vi "readPress02.vi"() -> ()   [LabVIEW 2011]
uses:
  Growth Sequences/Control 1.ctl
  <vilib>/Instr/_visa.llb/VISA Configure Serial Port (Instr).vi
panel:
  out "return count":u32
  in  "delay before read (ms)":u32=500
  in  "y":i32=1000
  in  "VISA resource name":T1="COM1"
  out "read buffer":string
  out "P (Torr)":dbl
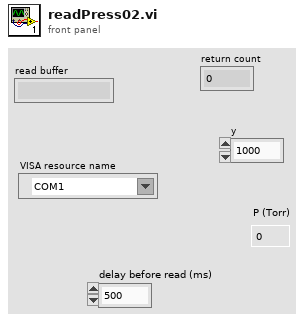
[diagram p1: front panel]
types:
  T1 = typedef "Control 1.ctl" = refnum<visa-resource-name>
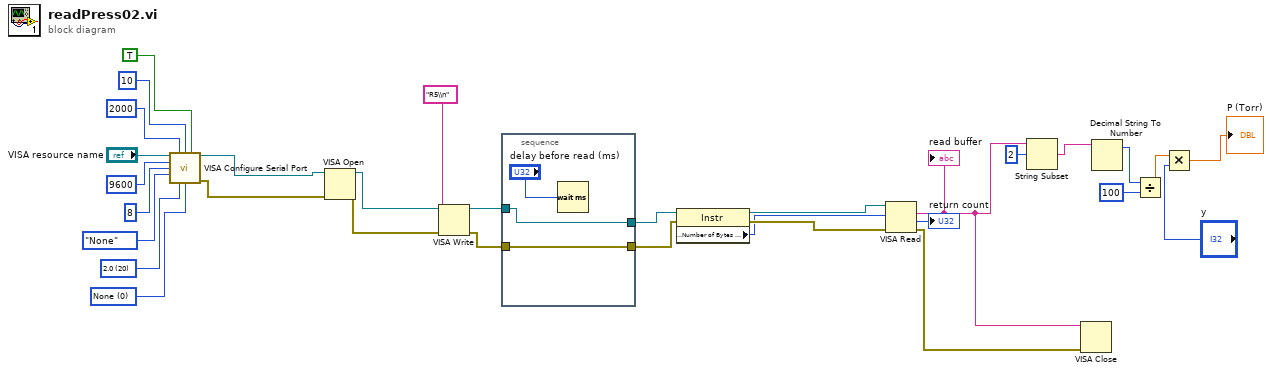
[diagram p0: block diagram]
diagram:
  w10 = u16 0 items=["None", "XON/XOFF", "RTS/CTS", "XON/XOFF & RTS/CTS", "DTR/DSR", "XON/XOFF & DTR/DSR"] ("flow control (0:none)")
  w11 = u16 20 items=["1.0"=10, "1.5"=15, "2.0"=20] ("stop bits (10: 1 bit)")
  n1 = call-poly "VISA Configure Serial Port"("VISA resource name"="VISA resource name", "timeout (10sec)"=u32 2000 ("General Settings:Timeout Value"), "termination char\n(0xA = '\\n' = LF)"=u8 10 ("termination char\n(0xA = '\\n' = LF)"), "Enable Termination\nChar (T)"=TRUE ("Enable Termination\nChar (T)"), "baud rate (9600)"=u32 9600, "data bits (8)"=u16 8, "parity (0:none)"=enum16{"None", "Odd", "Even", "Mark", "Space"}."None", "stop bits (10: 1 bit)"=w11, "flow control (0:none)"=w10) -> ("VISA resource name out"=w4:refnum<visa-resource-name>, "error out"=w3:errorcluster)  [unwired: 5 in]
  n2 = VISA Open(error in (no error)=w3, VISA resource name=w4) -> (VISA resource name=w2:refnum<visa-resource-name>, error out=w1:errorcluster)  [unwired: 3 in]
  n3 = VISA Write(VISA resource name=w2, write buffer="R5\\n", error in (no error)=w1) -> (VISA resource name out=w23:refnum<visa-resource-name>, error out=w22:errorcluster)  [unwired: 1 out]
  n4 = stacked-sequence {
    tunnel: w22 -> [w34]
    tunnel: [w34] -> w20
    tunnel: [w32] -> w21
    tunnel: w23 -> [w32]
    frame #0 {
      n5 = Wait (ms)(milliseconds to wait="delay before read (ms)") -> ()  [unwired: 1 out]
    }
  }
  n6 = property class="Instr"(reference=w21, error in=w20) -> (reference out=w18:refnum<visa-resource-name>, error out=w19:errorcluster, "Serial Settings:Number of Bytes at Serial Port"=w17:u32)
  n7 = VISA Read(VISA resource name=w18, byte count=w17, error in (no error)=w19) -> (read buffer=w7:string, return count=→"return count":u32, error out=w6:errorcluster)  [unwired: 1 out]
  "read buffer" <- w7
  n8 = String Subset(string=w7, offset (0)=2) -> (substring=w31:string)  [unwired: 1 in]
  n9 = VISA Close(VISA resource name=w7, error in (no error)=w6) -> ()  [unwired: 1 out]
  n10 = Decimal String To Number(string=w31) -> (offset past number=w26:i32)  [unwired: 2 in, 1 out]
  n11 = Divide(x=w26, y=100) -> (x/y=w24:dbl)
  n12 = Multiply(x=w24, y="y") -> (x*y=→"P (Torr)":dbl)
